vi "Test Server.vi"() -> ()   [LabVIEW 2013]
uses:
  lv-venv/lv.lib/vi.lib/LabVIEW Open Source Project/MQTT Control Packets/Control Packets/CONNACK/Connect Return Code -- enum.ctl
  lv-venv/lv.lib/vi.lib/LabVIEW Open Source Project/MQTT Control Packets/Control Packets/ControlPacket/QualityOfService -- enum.ctl
  source/MQTT_Server/Server class/Server.lvclass/Server.ctl
  <vilib>/LabVIEW Open Source Project/MQTT Client/Client class/Client.lvclass/Client.ctl
  lv-venv/lv.lib/vi.lib/LabVIEW Open Source Project/MQTT Control Packets/Control Packets/PUBLISH/PUBLISH.lvclass
  source/MQTT_Server/Server class/Server.lvclass
  <vilib>/LabVIEW Open Source Project/MQTT Connection/MQTT_Base/Base Class/MQTT_Base.lvclass
  <vilib>/LabVIEW Open Source Project/MQTT Client/Client class/Client.lvclass
  <vilib>/LabVIEW Open Source Project/MQTT TCP Connection/MQTT_TCP/Connection/TCPConnection.lvclass
  <vilib>/LabVIEW Open Source Project/MQTT LocalQueue Connection/MQTT_LocalQueue/Connection/LocalQueueConnection.lvclass
  <vilib>/LabVIEW Open Source Project/MQTT Websockets Connection/MQTT_Websockets/Connection/WebsocketsConnection.lvclass
  <vilib>/LabVIEW Open Source Project/MQTT Control Packets/Control Packets/CONNACK/CONNACK.lvclass
  <vilib>/LabVIEW Open Source Project/MQTT Control Packets/Control Packets/ControlPacket/ControlPacket.lvclass
panel:
  in  "QoS":T1
  out "Published":bool
  out "Unsuback received":bool
  out "Suback received":bool
  in  "Connection Type":enum16{"TCP", "Local Queue", "WebSockets"}(ring)
  out "error server":errorcluster
  in  "Unsubscribe":bool
  in  "Subscribe":bool
  out "error client sink 2":errorcluster
  out "Random 2":dbl(graph)
  out "received 2":i32
  out "received timer 2":u32
  out "Client Status 2":T2=enum."Server Unavailable"
  out "published timer":u32
  out "received timer":u32
  out "received":i32
  out "published":i32
  out "Random":dbl(graph)
  out "Client Status":T2=enum."Server Unavailable"
  out "error client source":errorcluster
  out "NbConnections":u32
  out "error client sink 1":errorcluster
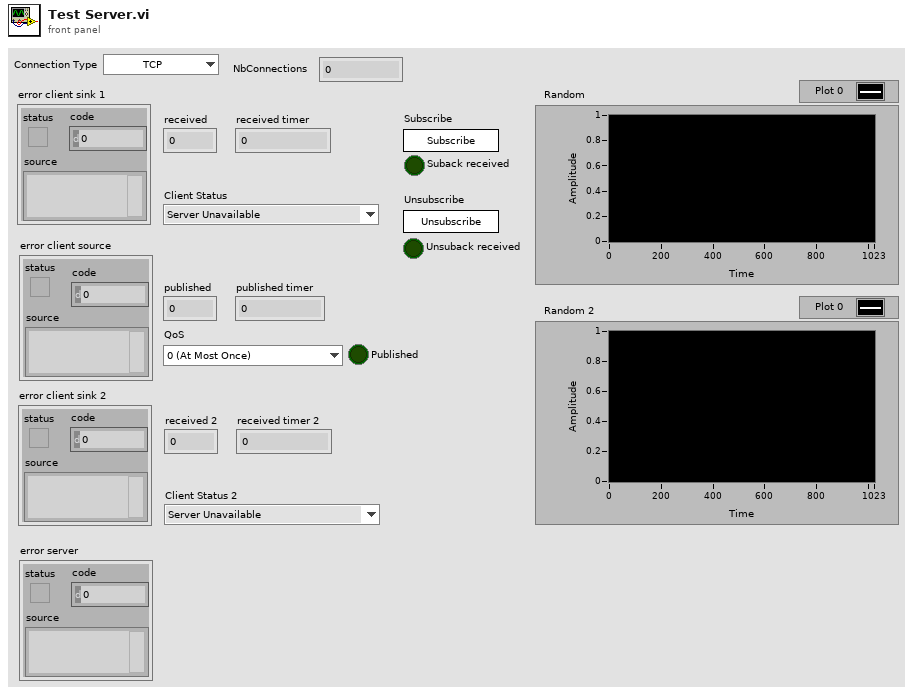
[diagram p1: front panel]
types:
  T1 = typedef "MQTT_Control_Packets.lvlib/ControlPacket.lvclass/QualityOfService -- enum.ctl" = enum16{"0 (At Most Once)", "1 (At Least Once)", "2 (Exactly Once)"}
  T2 = typedef "MQTT_Control_Packets.lvlib/CONNACK.lvclass/Connect Return Code -- enum.ctl" = enum16{"Connection accepted", "Unacceptable protocol version", "Identifier Rejected", "Server Unavailable", "Bad Username or Password", "Not Authorized"}
  T3 = typedef "MQTT Client.lvlib/Client.lvclass/Public Events -- cluster.ctl" = cluster{"Connection Status":refnum<user-event>, "Connected":refnum<user-event>, "Application Message":refnum<user-event>}
  T4 = typedef "MQTT Server.lvlib/Server.lvclass/Public Events -- cluster.ctl" = cluster{"NbConnections":refnum<user-event>}
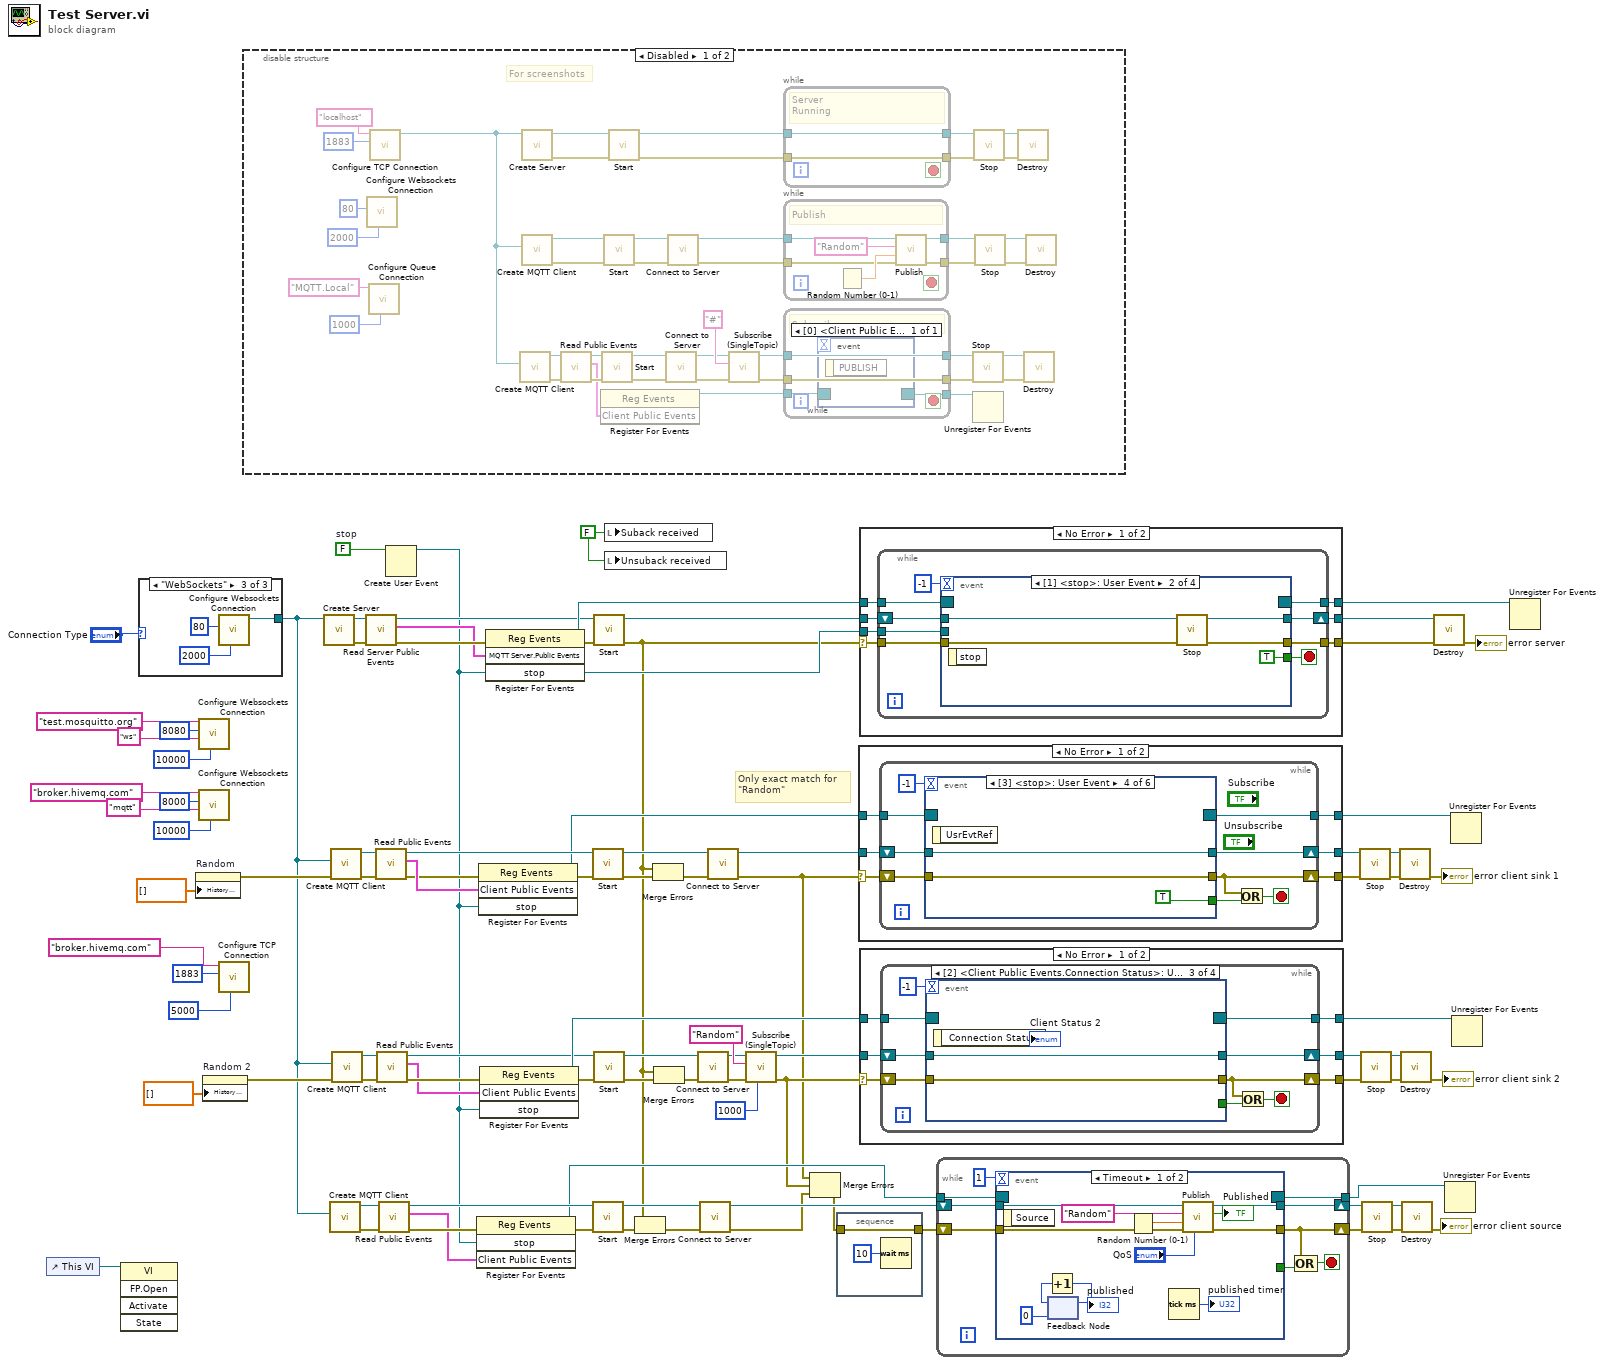
[diagram p0: block diagram]
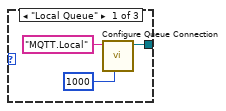
[diagram p2: hidden frame]
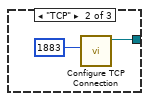
[diagram p3: hidden frame]
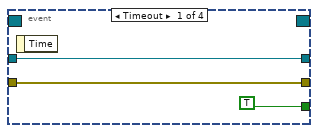
[diagram p5: hidden frame]
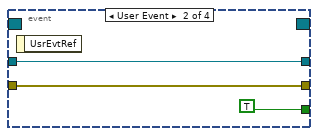
[diagram p6: hidden frame]
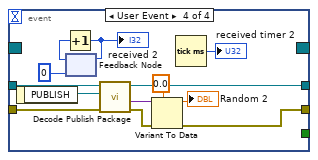
[diagram p7: hidden frame]
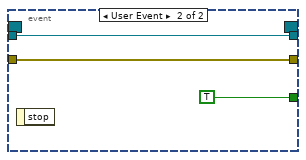
[diagram p9: hidden frame]
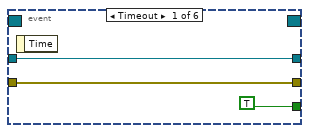
[diagram p10: hidden frame]
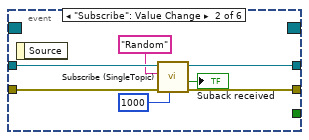
[diagram p11: hidden frame]
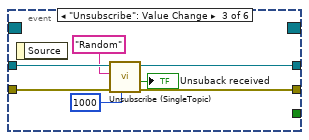
[diagram p12: hidden frame]
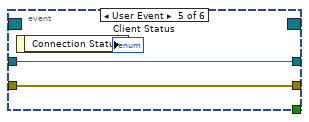
[diagram p13: hidden frame]
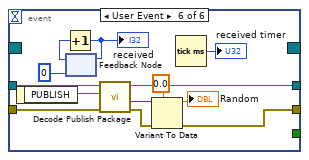
[diagram p14: hidden frame]
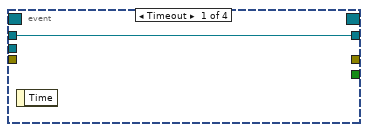
[diagram p16: hidden frame]
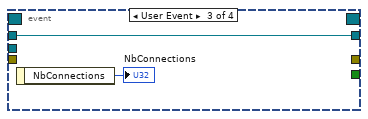
[diagram p17: hidden frame]
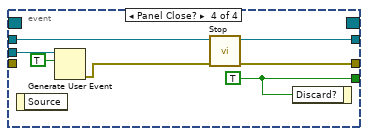
[diagram p18: hidden frame]
diagram:
  w14 = FALSE ("Suback received")
  w52 = FALSE  # stop
  # "Only exact match for\n\"Random\""
  n1 = control-ref of="This VI"() -> (w20:refnum<vi>)
  n2 = invoke class="VI" method="FP.Open"(reference=w20) -> ()  [unwired: 4 in, 5 out]
  n3 = case shown="\"WebSockets\"" "Connection Type" {
    tunnel: [w95 w98 w102] -> w1
    frame "Local Queue" {
      n4 = call "Configure Queue Connection.vi"("timeout (500 ms)"=1000 ("timeout (100ms)"), "Queue Name"="MQTT.Local") -> ("LocalQueueConnection"=w95:refnum<class "LocalQueueConnection.lvclass">)  [unwired: 8 in, 1 out]
    }
    frame "TCP" {
      n5 = call "Configure TCP Connection.vi"("remote port (80)"=u16 1883) -> ("TCPConnection"=w98:refnum<class "TCPConnection.lvclass">)  [unwired: 9 in, 1 out]
    }
    frame "WebSockets" {
      n6 = call "Configure Websockets Connection.vi"("timeout (5000 ms)"=2000 ("timeout (100ms)"), "remote port (80)"=u16 80) -> ("WSConnection"=w102:refnum<class "WebsocketsConnection.lvclass">)  [unwired: 8 in, 1 out]
    }
  }
  n7 = property on="Random" class="WFChart (strict)"("History Data"=dbl[] []) -> (error out=w56:errorcluster)  [unwired: 2 in, 1 out]
  n8 = call "Configure Websockets Connection.vi"("timeout (5000 ms)"=10000 ("timeout (100ms)"), "path"="ws", "remote port (80)"=u16 8080, "address (localhost)"="test.mosquitto.org") -> ()  [unwired: 6 in, 2 out]
  n9 = call "Configure Websockets Connection.vi"("timeout (5000 ms)"=10000 ("timeout (100ms)"), "path"="mqtt", "remote port (80)"=u16 8000, "address (localhost)"="broker.hivemq.com") -> ()  [unwired: 6 in, 2 out]
  n10 = property on="Random 2" class="WFChart (strict)"("History Data"=dbl[] []) -> (error out=w23:errorcluster)  [unwired: 2 in, 1 out]
  n11 = call "Configure TCP Connection.vi"("timeout (5000ms)"=5000 ("timeout (100ms)"), "remote port (80)"=u16 1883, "address (localhost)"="broker.hivemq.com") -> ()  [unwired: 7 in, 2 out]
  n12 = disable-structure shown="Disabled" {
    frame Disabled {
      # "For screenshots"
      n13 = call "Configure Websockets Connection.vi"("timeout (5000 ms)"=2000 ("timeout (100ms)"), "remote port (80)"=u16 80) -> ()  [unwired: 8 in, 2 out]
      n14 = call "Configure Queue Connection.vi"("timeout (500 ms)"=1000 ("timeout (100ms)"), "Queue Name"="MQTT.Local") -> ()  [unwired: 8 in, 2 out]
      n15 = call "Configure TCP Connection.vi"("remote port (80)"=u16 1883, "address (localhost)"="localhost" ("Topic Filter")) -> ("TCPConnection"=w108:refnum<class "TCPConnection.lvclass">)  [unwired: 8 in, 1 out]
      n16 = call <vilib>:"Create MQTT Client.vi"("Connection Configuration"=w108) -> ("error out"=w114:errorcluster, "Client out"=w116:refnum<class "Client.lvclass">)  [unwired: 9 in]
      n17 = call "Create Server.vi"("Connection Configuration"=w108) -> ("error out"=w139:errorcluster, "Server"=w138:refnum<class "Server.lvclass">)  [unwired: 9 in]
      n18 = call <vilib>:"Create MQTT Client.vi"("Connection Configuration"=w108) -> ("error out"=w136:errorcluster, "Client out"=w137:refnum<class "Client.lvclass">)  [unwired: 9 in]
      n19 = call <vilib>:"Read Public Events.vi"("error in (no error)"=w114, "Client in"=w116) -> ("error out"=w113:errorcluster, "Client Public Events"=w112:T3, "Client out"=w115:refnum<class "Client.lvclass">)  [unwired: 7 in]
      n20 = register-events(w112) -> (reference out=w111:refnum<event-registration>)  [unwired: 2 in, 1 out]
      n21 = call "Start.vi"("error in (no error)"=w113, "MQTT_Base in"=w115) -> ("error out"=w131:errorcluster, "MQTT_Base out"=w132:refnum<class "Client.lvclass">)  [unwired: 7 in, 1 out]
      n22 = call "Start.vi"("error in (no error)"=w136, "MQTT_Base in"=w137) -> ("error out"=w143:errorcluster, "MQTT_Base out"=w142:refnum<class "Client.lvclass">)  [unwired: 7 in, 1 out]
      n23 = call "Start.vi"("error in (no error)"=w139, "MQTT_Base in"=w138) -> ("error out"=w123:errorcluster, "MQTT_Base out"=w125:refnum<class "Server.lvclass">)  [unwired: 7 in, 1 out]
      n24 = call <vilib>:"Connect to Server.vi"("error in (no error)"=w131, "Client in"=w132) -> ("error out"=w119:errorcluster, "Client out"=w120:refnum<class "Client.lvclass">)  [unwired: 6 in, 2 out]
      n25 = call <vilib>:"Connect to Server.vi"("error in (no error)"=w143, "Client in"=w142) -> ("error out"=w127:errorcluster, "Client out"=w130:refnum<class "Client.lvclass">)  [unwired: 6 in, 2 out]
      n26 = call "Subscribe (SingleTopic).vi"("error in (no error)"=w119, "Topic Filter"="#", "MQTT_Base in"=w120) -> ("error out"=w117:errorcluster, "MQTT_Base out"=w118:refnum<class "Client.lvclass">)  [unwired: 6 in, 1 out]
      n27 = while {
        tunnel: [w157] -> w126
        tunnel: w125 -> [w157]
        tunnel: w123 -> [w156]
        tunnel: [w156] -> w124
        stop <- _ stop-if-true
        # "Server\nRunning"
      }
      n28 = while {
        tunnel: w130 -> [w153]
        tunnel: [w152] -> w129
        tunnel: [w151] -> w128
        tunnel: w127 -> [w150]
        stop <- _ stop-if-true
        # "Publish"
        n29 = Random Number (0-1)() -> (number: 0 to 1=w155:dbl)
        n30 = call <vilib>:"Publish.vi"("error in (no error)"=w150, "Payload"=w155, "Topic Name (empty: Payload name)"="Random", "Client in"=w153) -> ("error out"=w151:errorcluster, "Client out"=w152:refnum<class "Client.lvclass">)  [unwired: 5 in, 1 out]
      }
      n31 = while {
        tunnel: [w149] -> w121
        tunnel: w118 -> [w149]
        tunnel: w117 -> [w148]
        tunnel: [w148] -> w122
        tunnel: w111 -> [w147]
        tunnel: [w146] -> w110
        stop <- _ stop-if-true
        # "Subscribe"
        n32 = event shown="[0] <Client Public Events.Application Message>: User Event" {
          selector: w147 -> [_]
          dyn-events: [_] -> w146
          timeout: _ -> [_]
          event User Event {
            n33 = event-data() -> ()  [unwired: 1 in, 1 out]
          }
        }
      }
      n34 = call "Stop.vi"("error in (no error)"=w122, "MQTT_Base in"=w121) -> ("error out"=w134:errorcluster, "MQTT_Base out"=w135:refnum<class "Client.lvclass">)  [unwired: 7 in, 1 out]
      n35 = Unregister For Events(event registration refnum=w110) -> ()  [unwired: 1 in, 1 out]
      n36 = call "Stop.vi"("error in (no error)"=w124, "MQTT_Base in"=w126) -> ("error out"=w145:errorcluster, "MQTT_Base out"=w144:refnum<class "Server.lvclass">)  [unwired: 7 in, 1 out]
      n37 = call "Stop.vi"("error in (no error)"=w128, "MQTT_Base in"=w129) -> ("error out"=w141:errorcluster, "MQTT_Base out"=w140:refnum<class "Client.lvclass">)  [unwired: 7 in, 1 out]
      n38 = call "Destroy.vi"("error in (no error)"=w145, "MQTT_Base in"=w144) -> ()  [unwired: 8 in, 2 out]
      n39 = call "Destroy.vi"("error in (no error)"=w134, "MQTT_Base in"=w135) -> ()  [unwired: 8 in, 2 out]
      n40 = call "Destroy.vi"("error in (no error)"=w141, "MQTT_Base in"=w140) -> ()  [unwired: 8 in, 2 out]
    }
    frame Enabled {
    }
  }
  n41 = call "Create Server.vi"("Connection Configuration"=w1) -> ("error out"=w92:errorcluster, "Server"=w93:refnum<class "Server.lvclass">)  [unwired: 9 in]
  n42 = call <vilib>:"Create MQTT Client.vi"("Connection Configuration"=w1) -> ("error out"=w76:errorcluster, "Client out"=w75:refnum<class "Client.lvclass">)  [unwired: 9 in]
  n43 = call <vilib>:"Create MQTT Client.vi"("error in (no error)"=w56, "Connection Configuration"=w1) -> ("error out"=w77:errorcluster, "Client out"=w78:refnum<class "Client.lvclass">)  [unwired: 8 in]
  n44 = call <vilib>:"Create MQTT Client.vi"("error in (no error)"=w23, "Connection Configuration"=w1) -> ("error out"=w28:errorcluster, "Client out"=w27:refnum<class "Client.lvclass">)  [unwired: 8 in]
  n45 = call "Read Server Public Events.vi"("error in (no error)"=w92, "Server in"=w93) -> ("error out"=w91:errorcluster, "MQTT Server.Public Events"=w90:T4, "Server out"=w86:refnum<class "Server.lvclass">)  [unwired: 7 in]
  n46 = call <vilib>:"Read Public Events.vi"("error in (no error)"=w77, "Client in"=w78) -> ("error out"=w61:errorcluster, "Client Public Events"=w62:T3, "Client out"=w74:refnum<class "Client.lvclass">)  [unwired: 7 in]
  n47 = call <vilib>:"Read Public Events.vi"("error in (no error)"=w28, "Client in"=w27) -> ("error out"=w39:errorcluster, "Client Public Events"=w38:T3, "Client out"=w29:refnum<class "Client.lvclass">)  [unwired: 7 in]
  n48 = call <vilib>:"Read Public Events.vi"("error in (no error)"=w76, "Client in"=w75) -> ("error out"=w51:errorcluster, "Client Public Events"=w47:T3, "Client out"=w71:refnum<class "Client.lvclass">)  [unwired: 7 in]
  n49 = Create User Event(user event datatype=w52) -> (user event=w24:refnum<user-event>)  [unwired: 1 in, 1 out]
  n50 = register-events(error in=w51, w24, w47) -> (reference out=w49:refnum<event-registration>, error out=w50:errorcluster)  [unwired: 1 in]
  n51 = register-events(error in=w61, w62, w24) -> (reference out=w59:refnum<event-registration>, error out=w60:errorcluster)  [unwired: 1 in]
  n52 = register-events(error in=w39, w38, w24) -> (reference out=w41:refnum<event-registration>, error out=w40:errorcluster)  [unwired: 1 in]
  n53 = register-events(error in=w91, w90, w24) -> (reference out=w89:refnum<event-registration>, error out=w84:errorcluster)  [unwired: 1 in]
  n54 = call "Start.vi"("error in (no error)"=w60, "MQTT_Base in"=w74) -> ("error out"=w72:errorcluster, "MQTT_Base out"=w73:refnum<class "Client.lvclass">)  [unwired: 7 in, 1 out]
  n55 = call "Start.vi"("error in (no error)"=w50, "MQTT_Base in"=w71) -> ("error out"=w69:errorcluster, "MQTT_Base out"=w70:refnum<class "Client.lvclass">)  [unwired: 7 in, 1 out]
  n56 = call "Start.vi"("error in (no error)"=w84, "MQTT_Base in"=w86) -> ("error out"=w22:errorcluster, "MQTT_Base out"=w85:refnum<class "Server.lvclass">)  [unwired: 7 in, 1 out]
  n57 = call "Start.vi"("error in (no error)"=w40, "MQTT_Base in"=w29) -> ("error out"=w31:errorcluster, "MQTT_Base out"=w30:refnum<class "Client.lvclass">)  [unwired: 7 in, 1 out]
  n58 = local write "Suback received"(w14) -> ()
  n59 = local write "Unsuback received"(w14) -> ()
  n60 = Merge Errors(w22, w69) -> (w79:errorcluster)
  n61 = Merge Errors(w22, w72) -> (w80:errorcluster)
  n62 = Merge Errors(w22, w31) -> (w26:errorcluster)
  n63 = call <vilib>:"Connect to Server.vi"("error in (no error)"=w26, "Client in"=w30) -> ("error out"=w35:errorcluster, "Client out"=w34:refnum<class "Client.lvclass">)  [unwired: 6 in, 2 out]
  n64 = call <vilib>:"Connect to Server.vi"("error in (no error)"=w79, "Client in"=w70) -> ("error out"=w46:errorcluster, "Client out"=w87:refnum<class "Client.lvclass">)  [unwired: 6 in, 2 out]
  n65 = call <vilib>:"Connect to Server.vi"("error in (no error)"=w80, "Client in"=w73) -> ("error out"=w17:errorcluster, "Client out"=w18:refnum<class "Client.lvclass">)  [unwired: 6 in, 2 out]
  n66 = call "Subscribe (SingleTopic).vi"("timeout (100ms)"=1000, "error in (no error)"=w35, "Topic Filter"="Random", "MQTT_Base in"=w34) -> ("error out"=w21:errorcluster, "MQTT_Base out"=w43:refnum<class "Client.lvclass">)  [unwired: 5 in, 1 out]
  n67 = Merge Errors(w17, w21, w46) -> (w54:errorcluster)
  n68 = stacked-sequence {
    tunnel: [w158] -> w53
    tunnel: w54 -> [w158]
    frame #0 {
      n69 = Wait (ms)(milliseconds to wait=u32 10) -> ()  [unwired: 1 out]
    }
  }
  n70 = case shown="No Error" w17 {
    selector: w17 -> [w160 w211]
    tunnel: w59 -> [w165 w213]
    tunnel: [w164 w213] -> w58
    tunnel: w18 -> [w163 w212]
    tunnel: [w162 w212] -> w57
    tunnel: [w161 w211] -> w55
    frame No Error {
      n71 = while {
        tunnel: w165 -> [w174]
        tunnel: [w173] -> w164
        shift-right: [w171] -> w162
        shift-left: w163 -> [w172]
        shift-right: [w168] -> w161
        shift-left: w160 -> [w170]
        stop <- w169 stop-if-true
        n72 = event shown="[3] <stop>: User Event" {
          selector: w174 -> [_ _ _ _ _ _]
          dyn-events: [_ _ _ _ _ _] -> w173
          timeout: -1 -> [_ _ _ _ _ _]
          tunnel: w172 -> [w176 w184 w191 w193 w196 w209]
          tunnel: [w176 w181 w190 w193 w196 w205] -> w171
          tunnel: [w175 w180 w187 w192 w195 w198] -> w168
          tunnel: w170 -> [w175 w183 w188 w192 w195 w204]
          tunnel: [TRUE _ _ TRUE _ _] -> w167
          event Timeout {
            n73 = event-data() -> ()  [unwired: 1 in, 1 out]
          }
          event "Subscribe": Value Change {
            n74 = event-data() -> ()  [unwired: 1 in, 1 out]
            n75 = call "Subscribe (SingleTopic).vi"("timeout (100ms)"=1000, "error in (no error)"=w183, "Topic Filter"="Random", "MQTT_Base in"=w184) -> ("error out"=w180:errorcluster, "Ack"=→"Suback received":bool, "MQTT_Base out"=w181:refnum<class "Client.lvclass">)  [unwired: 5 in]
          }
          event "Unsubscribe": Value Change {
            n76 = event-data() -> ()  [unwired: 1 in, 1 out]
            n77 = call "Unsubscribe (SingleTopic).vi"("timeout (100ms)"=1000, "error in (no error)"=w188, "Topic Filter"="Random", "MQTT_Base in"=w191) -> ("error out"=w187:errorcluster, "Ack"=→"Unsuback received":bool, "MQTT_Base out"=w190:refnum<class "Client.lvclass">)  [unwired: 5 in]
          }
          event User Event {
            n78 = event-data() -> ()  [unwired: 1 in, 1 out]
          }
          event User Event {
            n79 = event-data() -> ("Connection Status"=→"Client Status":T2)  [unwired: 1 in]
          }
          event User Event {
            n80 = event-data() -> ("PUBLISH"=w210:refnum<class "PUBLISH.lvclass">)  [unwired: 1 in]
            n81 = feedback #1(0 ("received")) -> (w202:i32)
            n82 = Increment(x=w202) -> (x+1=w201:i32)
            "received" <- w201
            n83 = feedback-in #1(w201) -> ()
            n84 = call "Decode Publish Package.vi"("error in (no error)"=w204, "PUBLISH in"=w210, "MQTT_Base in"=w209) -> ("error out"=w199:errorcluster, "Payload"=w208:variant, "MQTT_Base out"=w205:refnum<class "Client.lvclass">)  [unwired: 5 in, 1 out]
            n85 = Variant To Data(error in=w199, type=0.0, Variant=w208) -> (data=→"Random":dbl, error out=w198:errorcluster)
            n86 = Tick Count (ms)() -> (millisecond timer value=→"received timer":u32)
          }
        }
        n87 = Or(x=w168, y=w167) -> (x .or. y?=w169:bool)
      }
    }
    frame Error {
    }
  }
  n88 = case shown="No Error" w22 {
    selector: w22 -> [w214 w245]
    tunnel: w85 -> [w220 w247]
    tunnel: [w219 w247] -> w94
    tunnel: w89 -> [w218 w246]
    tunnel: [w217 w246] -> w88
    tunnel: [w216 w245] -> w83
    tunnel: w24 -> [w215 _]
    frame No Error {
      n89 = while {
        shift-right: [w226] -> w219
        shift-left: w220 -> [w228]
        tunnel: w218 -> [w225]
        tunnel: [w224] -> w217
        tunnel: [w223] -> w216
        tunnel: w215 -> [w222]
        tunnel: w214 -> [w221]
        stop <- w227 stop-if-true
        n90 = event shown="[1] <stop>: User Event" {
          selector: w225 -> [_ _ _ _]
          dyn-events: [_ _ _ _] -> w224
          timeout: -1 -> [_ _ _ _]
          tunnel: w228 -> [w230 w235 w237 w244]
          tunnel: [_ TRUE ("Discard?") _ w243] -> w227
          tunnel: [w230 w234 w237 w242] -> w226
          tunnel: [_ w233 _ w241] -> w223
          tunnel: w222 -> [_ _ _ w240]
          tunnel: w221 -> [_ w231 _ _]
          event Timeout {
            n91 = event-data() -> ()  [unwired: 1 in, 1 out]
          }
          event User Event {
            n92 = event-data() -> ()  [unwired: 1 in, 1 out]
            n93 = call "Stop.vi"("error in (no error)"=w231, "MQTT_Base in"=w235) -> ("error out"=w233:errorcluster, "MQTT_Base out"=w234:refnum<class "Server.lvclass">)  [unwired: 7 in, 1 out]
          }
          event User Event {
            n94 = event-data() -> ("NbConnections"=→"NbConnections":u32)  [unwired: 1 in]
          }
          event Panel Close? {
            w243 = TRUE ("Discard?")
            n95 = event-data() -> ()  [unwired: 1 in, 1 out]
            n96 = Generate User Event(user event=w240, event data cluster=TRUE ("event data")) -> (error out=w238:errorcluster)  [unwired: 2 in, 1 out]
            n97 = call "Stop.vi"("error in (no error)"=w238, "MQTT_Base in"=w244) -> ("error out"=w241:errorcluster, "MQTT_Base out"=w242:refnum<class "Server.lvclass">)  [unwired: 7 in, 1 out]
            n98 = event-data("Discard?"=w243) -> ()  [unwired: 1 in, 1 out]
          }
        }
      }
    }
    frame Error {
    }
  }
  n99 = case shown="No Error" w21 {
    selector: w21 -> [w248 w285]
    tunnel: w41 -> [w253 w287]
    tunnel: [w252 w287] -> w42
    tunnel: w43 -> [w251 w286]
    tunnel: [w250 w286] -> w44
    tunnel: [w249 w285] -> w45
    frame No Error {
      n100 = while {
        tunnel: w253 -> [w262]
        tunnel: [w261] -> w252
        shift-right: [w259] -> w250
        shift-left: w251 -> [w260]
        shift-right: [w256] -> w249
        shift-left: w248 -> [w258]
        stop <- w257 stop-if-true
        n101 = event shown="[2] <Client Public Events.Connection Status>: User Event" {
          selector: w262 -> [_ _ _ _]
          dyn-events: [_ _ _ _] -> w261
          timeout: -1 -> [_ _ _ _]
          tunnel: w260 -> [w264 w267 w270 w283]
          tunnel: [w264 w267 w270 w279] -> w259
          tunnel: [w263 w266 w269 w272] -> w256
          tunnel: w258 -> [w263 w266 w269 w278]
          tunnel: [TRUE TRUE _ _] -> w255
          event Timeout {
            n102 = event-data() -> ()  [unwired: 1 in, 1 out]
          }
          event User Event {
            n103 = event-data() -> ()  [unwired: 1 in, 1 out]
          }
          event User Event {
            n104 = event-data() -> ("Connection Status"=→"Client Status 2":T2)  [unwired: 1 in]
          }
          event User Event {
            n105 = event-data() -> ("PUBLISH"=w284:refnum<class "PUBLISH.lvclass">)  [unwired: 1 in]
            n106 = feedback #2(0 ("received")) -> (w276:i32)
            n107 = Increment(x=w276) -> (x+1=w275:i32)
            "received 2" <- w275
            n108 = feedback-in #2(w275) -> ()
            n109 = call "Decode Publish Package.vi"("error in (no error)"=w278, "PUBLISH in"=w284, "MQTT_Base in"=w283) -> ("error out"=w273:errorcluster, "Payload"=w282:variant, "MQTT_Base out"=w279:refnum<class "Client.lvclass">)  [unwired: 5 in, 1 out]
            n110 = Variant To Data(error in=w273, type=0.0, Variant=w282) -> (data=→"Random 2":dbl, error out=w272:errorcluster)
            n111 = Tick Count (ms)() -> (millisecond timer value=→"received timer 2":u32)
          }
        }
        n112 = Or(x=w256, y=w255) -> (x .or. y?=w257:bool)
      }
    }
    frame Error {
    }
  }
  n113 = while {
    shift-right: [w295] -> w68
    shift-left: w87 -> [w296]
    shift-right: [w288] -> w48
    shift-left: w53 -> [w294]
    tunnel: w49 -> [w292]
    tunnel: [w290] -> w19
    stop <- w293 stop-if-true
    n114 = event shown="[0] Timeout" {
      selector: w292 -> [_ _]
      dyn-events: [_ _] -> w290
      timeout: 1 -> [_ _]
      tunnel: w296 -> [w304 w309]
      tunnel: [w303 w309] -> w295
      tunnel: w294 -> [w302 w310]
      tunnel: [w301 w310] -> w288
      tunnel: [_ TRUE] -> w291
      event Timeout {
        n115 = event-data() -> ()  [unwired: 1 in, 1 out]
        n116 = feedback #3(0 ("received")) -> (w307:i32)
        n117 = Increment(x=w307) -> (x+1=w305:i32)
        "published" <- w305
        n118 = feedback-in #3(w305) -> ()
        n119 = Random Number (0-1)() -> (number: 0 to 1=w299:dbl)
        n120 = Tick Count (ms)() -> (millisecond timer value=→"published timer":u32)
        n121 = call <vilib>:"Publish.vi"("QoS"="QoS", "error in (no error)"=w302, "Payload"=w299, "Topic Name (empty: Payload name)"="Random", "Client in"=w304) -> ("error out"=w301:errorcluster, "Published"=→"Published":bool, "Client out"=w303:refnum<class "Client.lvclass">)  [unwired: 4 in]
      }
      event User Event {
        n122 = event-data() -> ()  [unwired: 1 in, 1 out]
      }
    }
    n123 = Compound Arithmetic op=OR(w288, w291) -> (w293:bool)
  }
  n124 = call "Stop.vi"("error in (no error)"=w55, "MQTT_Base in"=w57) -> ("error out"=w65:errorcluster, "MQTT_Base out"=w64:refnum<class "Client.lvclass">)  [unwired: 7 in, 1 out]
  n125 = call "Stop.vi"("error in (no error)"=w45, "MQTT_Base in"=w44) -> ("error out"=w32:errorcluster, "MQTT_Base out"=w33:refnum<class "Client.lvclass">)  [unwired: 7 in, 1 out]
  n126 = call "Stop.vi"("error in (no error)"=w48, "MQTT_Base in"=w68) -> ("error out"=w66:errorcluster, "MQTT_Base out"=w67:refnum<class "Client.lvclass">)  [unwired: 7 in, 1 out]
  n127 = call "Destroy.vi"("error in (no error)"=w65, "MQTT_Base in"=w64) -> ("error out"=→"error client sink 1":errorcluster)  [unwired: 8 in, 1 out]
  n128 = call "Destroy.vi"("error in (no error)"=w32, "MQTT_Base in"=w33) -> ("error out"=→"error client sink 2":errorcluster)  [unwired: 8 in, 1 out]
  n129 = call "Destroy.vi"("error in (no error)"=w66, "MQTT_Base in"=w67) -> ("error out"=→"error client source":errorcluster)  [unwired: 8 in, 1 out]
  n130 = call "Destroy.vi"("error in (no error)"=w83, "MQTT_Base in"=w94) -> ("error out"=→"error server":errorcluster)  [unwired: 8 in, 1 out]
  n131 = Unregister For Events(event registration refnum=w19) -> ()  [unwired: 1 in, 1 out]
  n132 = Unregister For Events(event registration refnum=w58) -> ()  [unwired: 1 in, 1 out]
  n133 = Unregister For Events(event registration refnum=w42) -> ()  [unwired: 1 in, 1 out]
  n134 = Unregister For Events(event registration refnum=w88) -> ()  [unwired: 1 in, 1 out]
